vi "Truncate string.vi"(11 "File Path":path) -> (3 "String path out":string)   [LabVIEW 2020]
doc: "Trunctates a path string so that the display only contains a designated number of characters.\n\nLength is currently limited to 35 characters."
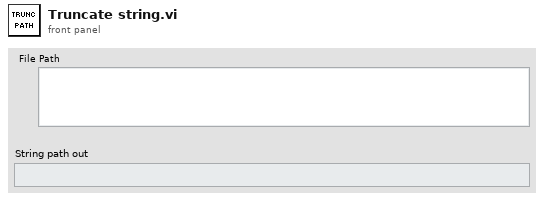
[diagram p1: front panel]
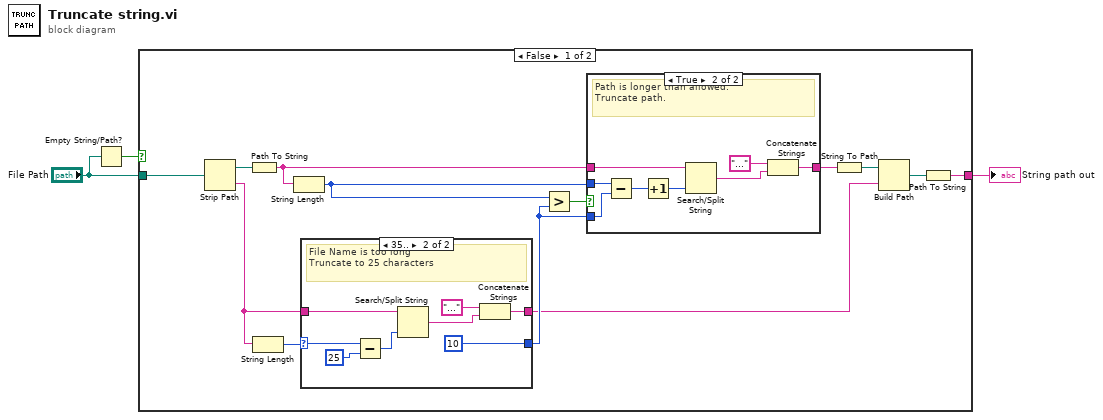
[diagram p0: block diagram]
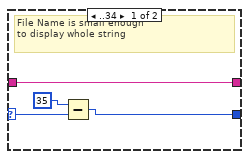
[diagram p2: hidden frame]
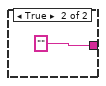
[diagram p4: hidden frame]
diagram:
  n1 = Empty String/Path?(string/path="File Path") -> (empty?=w3:bool)
  n2 = case shown="False" w3 {
    tunnel: [w8 ""] -> w1
    tunnel: "File Path" -> [w4 _]
    frame False {
      n3 = Strip Path(path=w4) -> (stripped path=w13:path, name=w6:string)
      n4 = Path To String(path=w13) -> (string=w12:string)
      n5 = String Length(string=w6) -> (length=w7:i32)
      n6 = String Length(string=w12) -> (length=w15:i32)
      n7 = case shown="35.." w7 {
        selector: w7 -> [w18 w23]
        tunnel: [w19 10] -> w14
        tunnel: w6 -> [w17 w27]
        tunnel: [w17 w24] -> w5
        frame ..34 {
          # "File Name is small enough\nto display whole string"
          n8 = Subtract(x=35 ("length"), y=w18) -> (x-y=w19:i32)
        }
        frame 35.. {
          # "File Name is too long\nTruncate to 25 characters"
          n9 = Subtract(x=w23, y=25) -> (x-y=w21:i32)
          n10 = Search/Split String(string=w27, offset (0)=w21) -> (match + rest of string=w25:string)  [unwired: 3 out]
          n11 = Concatenate Strings("..." ("string"), w25) -> (w24:string)
        }
      }
      n12 = Greater?(x=w15, y=w14) -> (0:w16:bool)
      n13 = case shown="True" w16 {
        tunnel: w15 -> [_ w37]
        tunnel: w12 -> [w29 w33]
        tunnel: w14 -> [_ w36]
        tunnel: [w29 w34] -> w11
        frame False {
          # "Path is short enough."
        }
        frame True {
          # "Path is longer than allowed.\nTruncate path."
          n14 = Subtract(x=w37, y=w36) -> (x-y=w31:i32)
          n15 = Increment(x=w31) -> (x+1=w30:i32)
          n16 = Search/Split String(string=w33, offset (0)=w30) -> (match + rest of string=w32:string)  [unwired: 3 out]
          n17 = Concatenate Strings("..." ("string"), w32) -> (w34:string)
        }
      }
      n18 = String To Path(string=w11) -> (path=w10:path)
      n19 = Build Path(base path=w10, name or relative path=w5) -> (appended path=w9:path)
      n20 = Path To String(path=w9) -> (string=w8:string)
    }
    frame True {
    }
  }
  "String path out" <- w1
